vi "Glyph_MouseDown.vi"(6 "Double Click":bool, 8 "error in":errorcluster, 9 "Coords":T5, 10 "CtlRef":refnum<vi>, 11 "Data in":T1={"Class"={"Ants"=refnum, "Layer"=refnum, "Templates"=refnum, "Icon"=refnum, "Glyph"=refnum, "Settings"=refnum, "Tools"=refnum}, "Ref"={"Add Layer"=refnum, "Remove Layer"=refnum, "Line Text"=[], "Body Text Spec"=refnum, "DNL_Font"=refnum, "glyph path str"=refnum, "templates path str"=refnum, "Arrow Up"=refnum, "Arrow Down"=refnum, "IE VI Ref"=refnum, "Glyphs tree"=refnum, "Templates tree"=refnum, "Layer Icon Text"=refnum, "Layer Template"=refnum, "Body Text"=refnum, "Search Templates"=refnum, "TextMarker"=refnum, "Tab Control"=refnum, "Search Glyphs"=refnum, "Line Color"=refnum, "DNL_Glyphs []"=refnum, "Fill Color"=refnum, "Tools"=refnum, "Icon"=refnum, "Preview"=refnum, "Ants"=refnum, "Terminals"=refnum, "menu reference"=refnum, "LayerNames"=[], "GlyphLoadAnimation"=refnum, "TemplateLoadAnimation"=refnum, "refreshGlyphs"=refnum, "refreshTemplates"=refnum}, "Support"={"AntsRect"={"left"=0, "top"=0, "right"=0, "bottom"=0}, "Mouse Move Coords"={"Horizontal"=0, "Vertical"=0}, "Mouse Down Coords"={"Horizontal"=0, "Vertical"=0}, "Temp Coord"={"Horizontal"=0, "Vertical"=0}, "Action"=enum."Default", "Edge Color"=4914962, "Fill Color"=16860, "Mouse Down?"=FALSE, "Draft Mode?"=FALSE, "Temp Icon"=bytes[3102], "CTRL Pressed"=FALSE, "Move Selection?"=FALSE, "AntsRect Orig"={"left"=0, "top"=0, "right"=0, "bottom"=0}, "Text"="", "TM Set?"=FALSE, "Mouse inside icon?"=FALSE, "Tool (old value)"=0, "Pencil Move Color"=0, "Swap Colors?"=FALSE, "Shift pressed?"=FALSE}}) -> (0 "error out":errorcluster, 3 "Data out":T1={"Class"={"Ants"=refnum, "Layer"=refnum, "Templates"=refnum, "Icon"=refnum, "Glyph"=refnum, "Settings"=refnum, "Tools"=refnum}, "Ref"={"Add Layer"=refnum, "Remove Layer"=refnum, "Line Text"=[], "Body Text Spec"=refnum, "DNL_Font"=refnum, "glyph path str"=refnum, "templates path str"=refnum, "Arrow Up"=refnum, "Arrow Down"=refnum, "IE VI Ref"=refnum, "Glyphs tree"=refnum, "Templates tree"=refnum, "Layer Icon Text"=refnum, "Layer Template"=refnum, "Body Text"=refnum, "Search Templates"=refnum, "TextMarker"=refnum, "Tab Control"=refnum, "Search Glyphs"=refnum, "Line Color"=refnum, "DNL_Glyphs []"=refnum, "Fill Color"=refnum, "Tools"=refnum, "Icon"=refnum, "Preview"=refnum, "Ants"=refnum, "Terminals"=refnum, "menu reference"=refnum, "LayerNames"=[], "GlyphLoadAnimation"=refnum, "TemplateLoadAnimation"=refnum, "refreshGlyphs"=refnum, "refreshTemplates"=refnum}, "Support"={"AntsRect"={"left"=0, "top"=0, "right"=0, "bottom"=0}, "Mouse Move Coords"={"Horizontal"=0, "Vertical"=0}, "Mouse Down Coords"={"Horizontal"=0, "Vertical"=0}, "Temp Coord"={"Horizontal"=0, "Vertical"=0}, "Action"=enum."Default", "Edge Color"=4914962, "Fill Color"=16860, "Mouse Down?"=FALSE, "Draft Mode?"=FALSE, "Temp Icon"=bytes[3102], "CTRL Pressed"=FALSE, "Move Selection?"=FALSE, "AntsRect Orig"={"left"=0, "top"=0, "right"=0, "bottom"=0}, "Text"="", "TM Set?"=FALSE, "Mouse inside icon?"=FALSE, "Tool (old value)"=0, "Pencil Move Color"=0, "Swap Colors?"=FALSE, "Shift pressed?"=FALSE}})   [LabVIEW 2021]
uses:
  <vilib>/LabVIEW Icon API/lv_icon/Controls/Graphic.ctl
  <vilib>/Utility/miscctls.llb/LVPoint32TypeDef.ctl
  <resource>/plugins/NIIconEditor/Controls/Global Data.ctl
  <resource>/plugins/NIIconEditor/Class/Ants/Ants.lvclass
  <resource>/plugins/NIIconEditor/Class/FakedArray/FakedArray.lvclass
  <vilib>/LabVIEW Icon API/lv_icon/Classes/Icon/Icon.lvclass
  <resource>/plugins/NIIconEditor/Class/Icon Library/Glyph.lvclass
  <resource>/plugins/NIIconEditor/Class/Settings/Settings.lvclass
  <resource>/plugins/NIIconEditor/Class/Tools/Tools Paint.lvclass
  <resource>/plugins/NIIconEditor/Controls/IE Classes.ctl
  <resource>/plugins/NIIconEditor/Controls/References Cluster.ctl
  <resource>/plugins/NIIconEditor/Controls/SupportClass.ctl
  <resource>/plugins/NIIconEditor/Controls/SupportClass_Action.ctl
  <vilib>/LabVIEW Icon API/lv_icon/Controls/IEColor.ctl
  <resource>/plugins/NIIconEditor/Controls/Tools.ctl
  <vilib>/LabVIEW Icon API/lv_icon/lv_icon.lvlib
panel:
  in  "Path & Icon 2":T8
  in  "Path & Icon":T8
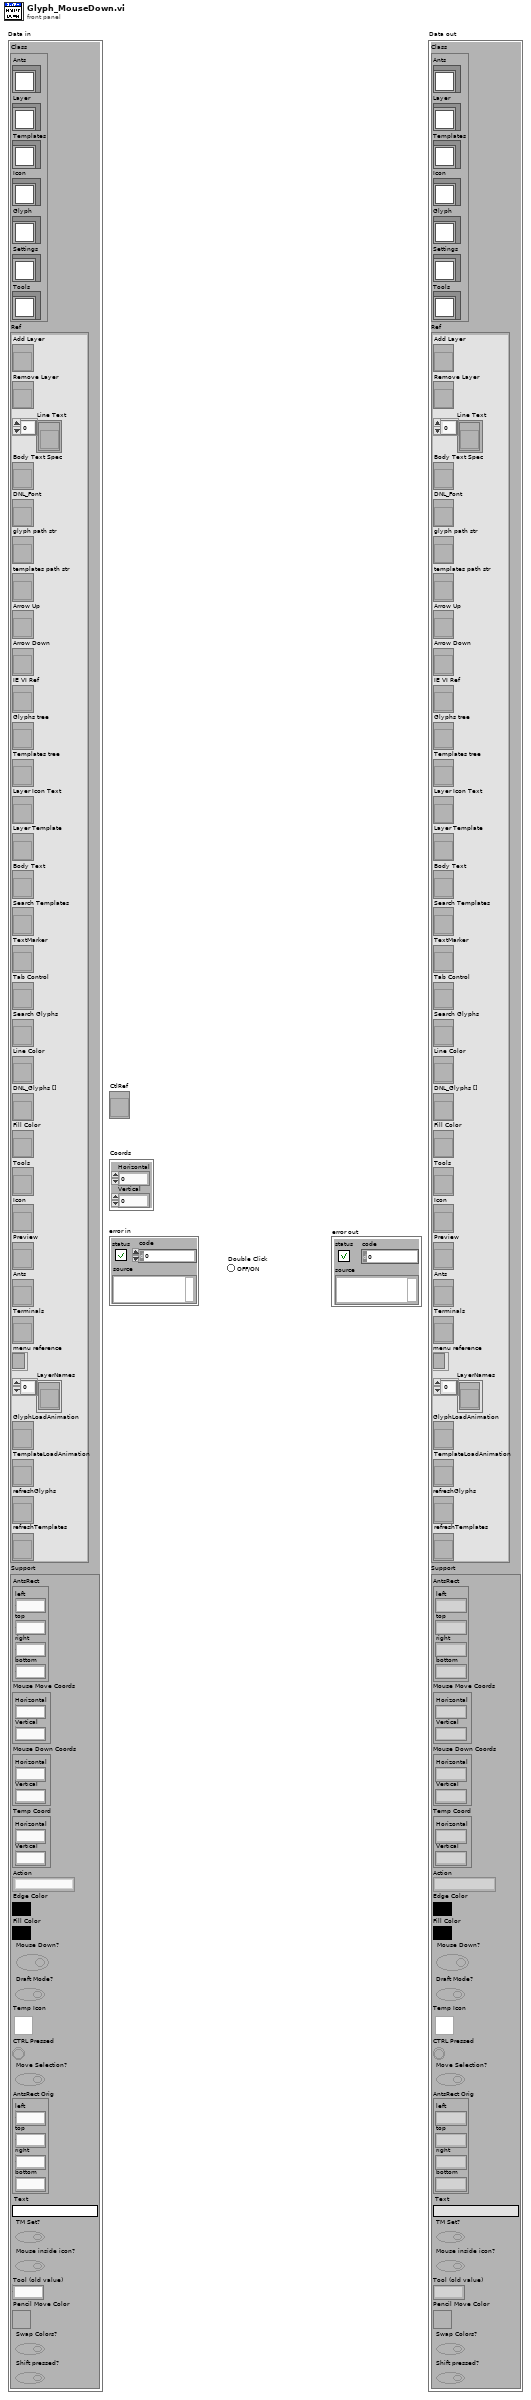
[diagram p1: front panel]
types:
  T1 = typedef "lv_icon.lvlib/Global Data.ctl" = cluster{"Class":T2, "Ref":T3, "Support":T4}
  T2 = typedef "IE Classes.ctl" = cluster{"Ants":refnum<class "Ants.lvclass">, "Layer":refnum<class "FakedArray.lvclass">, "Templates":refnum<class "FakedArray.lvclass">, "Icon":refnum<class "Icon.lvclass">, "Glyph":refnum<class "Glyph.lvclass">, "Settings":refnum<class "Settings.lvclass">, "Tools":refnum<class "Tools Paint.lvclass">}
  T3 = typedef "lv_icon.lvlib/References Cluster.ctl" = cluster{"Add Layer":refnum<vi>, "Remove Layer":refnum<vi>, "Line Text":refnum<vi>[], "Body Text Spec":refnum<vi>, "DNL_Font":refnum<vi>, "glyph path str":refnum<vi>, "templates path str":refnum<vi>, "Arrow Up":refnum<vi>, "Arrow Down":refnum<vi>, "IE VI Ref":refnum<vi>, "Glyphs tree":refnum<vi>, "Templates tree":refnum<vi>, "Layer Icon Text":refnum<vi>, "Layer Template":refnum<vi>, "Body Text":refnum<vi>, "Search Templates":refnum<vi>, "TextMarker":refnum<vi>, "Tab Control":refnum<vi>, "Search Glyphs":refnum<vi>, "Line Color":refnum<vi>, "DNL_Glyphs []":refnum<vi>, "Fill Color":refnum<vi>, "Tools":refnum<vi>, "Icon":refnum<vi>, "Preview":refnum<vi>, "Ants":refnum<vi>, "Terminals":refnum<vi>, "menu reference":refnum<k9>, "LayerNames":refnum<vi>[], "GlyphLoadAnimation":refnum<vi>, "TemplateLoadAnimation":refnum<vi>, "refreshGlyphs":refnum<vi>, "refreshTemplates":refnum<vi>}
  T4 = typedef "SupportClass.ctl" = cluster{"AntsRect":cluster{"left":i16, "top":i16, "right":i16, "bottom":i16}, "Mouse Move Coords":T5, "Mouse Down Coords":T5, "Temp Coord":T5, "Action":T6, "Edge Color":T7, "Fill Color":T7, "Mouse Down?":bool, "Draft Mode?":bool, "Temp Icon":picture, "CTRL Pressed":bool, "Move Selection?":bool, "AntsRect Orig":cluster{"left":i16, "top":i16, "right":i16, "bottom":i16}, "Text":string, "TM Set?":bool, "Mouse inside icon?":bool, "Tool (old value)":u32, "Pencil Move Color":u32, "Swap Colors?":bool, "Shift pressed?":bool}
  T5 = typedef "LVPoint32TypeDef.ctl" = cluster{"Horizontal":i32, "Vertical":i32}
  T6 = typedef "SupportClass_Action.ctl" = enum16{"Default", "Move Selection", "Glyph Library", "Tool"}
  T7 = typedef "IEColor.ctl" = u32
  T8 = typedef "Graphic.ctl" = cluster{"Rectangle":cluster{"left":i16, "top":i16, "right":i16, "bottom":i16}, "Path":path, "Image":picture, "Filter":string, "FileName":string}
  T9 = typedef "Tools.ctl" = enum32{"Pencil", "Line", "Dropper", "Fill", "Rectangle", "Filled Rectangle", "Ellipse", "Filled Ellipse", "Eraser", "Text", "Select", "Move"}
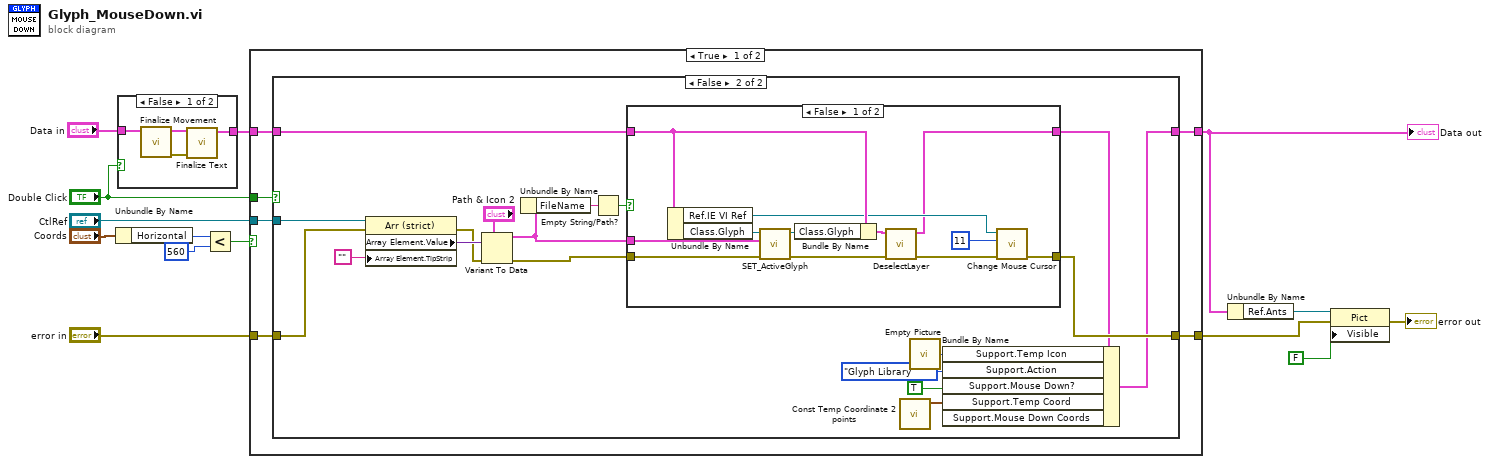
[diagram p0: block diagram]
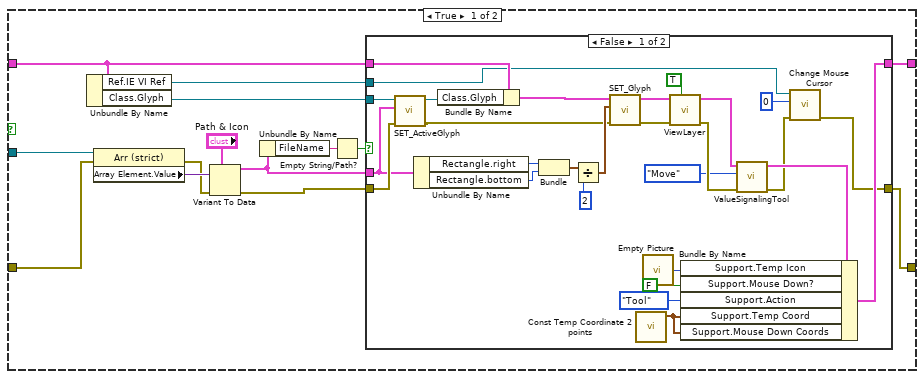
[diagram p3: hidden frame]
diagram:
  n1 = Unbundle By Name("Coords") -> ("Horizontal"=w6:i32)
  n2 = case shown="False" "Double Click" {
    tunnel: "Data in" -> [w17 w19]
    tunnel: [w15 w19] -> w4
    frame False {
      n3 = call <resource>:"Finalize Movement.vi"("Data in"=w17) -> ("error out"=w18:errorcluster, "Data out"=w16:T1)  [unwired: 2 in, 7 out]
      n4 = call <resource>:"Finalize Text.vi"("error in (no error)"=w18, "Data in"=w16) -> ("Data out"=w15:T1)  [unwired: 9 out]
    }
    frame True {
    }
  }
  n5 = Less?(x=w6, y=560 ("x")) -> (x < y?=w8:bool)
  n6 = case shown="True" w8 {
    tunnel: "CtlRef" -> [w25 _]
    tunnel: "error in" -> [w24 w103]
    tunnel: [w23 w103] -> w1
    tunnel: "Double Click" -> [w22 _]
    tunnel: w4 -> [w21 w102]
    tunnel: [w20 w102] -> w2
    frame True {
      n7 = case shown="False" w22 {
        tunnel: w25 -> [w39 w87]
        tunnel: w24 -> [w34 w83]
        tunnel: [w29 w77] -> w23
        tunnel: w21 -> [w32 w75]
        tunnel: [w31 w73] -> w20
        frame True {
          n8 = Unbundle By Name(w32) -> ("Ref.IE VI Ref"=w30:refnum<vi>, "Class.Glyph"=w33:refnum<class "Glyph.lvclass">)
          n9 = property class="Arr (strict)"(reference=w39, error in=w34) -> (error out=w37:errorcluster, "Array Element.Value"=w38:variant)  [unwired: 1 out]
          n10 = Variant To Data(error in=w37, type="Path & Icon", Variant=w38) -> (data=w27:T8, error out=w35:errorcluster)
          n11 = Unbundle By Name(w27) -> ("FileName"=w28:string)
          n12 = Empty String/Path?(string/path=w28) -> (empty?=w26:bool)
          n13 = case shown="False" w26 {
            tunnel: w35 -> [w67 w68]
            tunnel: w33 -> [w54 _]
            tunnel: w32 -> [w51 w69]
            tunnel: [w50 w69] -> w31
            tunnel: w30 -> [w43 _]
            tunnel: [w41 w68] -> w29
            tunnel: w27 -> [w40 _]
            frame False {
              n14 = call-dynamic "SET_ActiveGlyph.vi"("error in (no error)"=w67, "Active Glyph"=w40, "Glyph in"=w54) -> ("error out"=w52:errorcluster, "Glyph out"=w53:refnum<class "Glyph.lvclass">)  [unwired: 7 out]
              n15 = Unbundle By Name(w40) -> ("Rectangle.right"=w66:i16, "Rectangle.bottom"=w65:i16)
              n16 = Bundle By Name(cluster=w51, "Class.Glyph"=w53) -> (w49:T1)
              n17 = Bundle("right"=w66, "bottom"=w65) -> (w64:cluster{"right":i16, "bottom":i16})  [unwired: 1 out]
              n18 = Divide(x=w64, y=2) -> (x/y=w62:cluster{"right":dbl, "bottom":dbl})
              n19 = call <resource>:"SET_Glyph.vi"("error in"=w52, "Coordinates"=w62, "Data in"=w49) -> ("error out"=w56:errorcluster, "Data out"=w48:T1)  [unwired: 7 out]
              n20 = call <resource>:"Const Temp Coordinate 2 points.vi"() -> ("Const Temp Coordinate"=w58:T5)  [unwired: 11 out]
              n21 = call "Empty Picture"() -> ("empty picture"=w59:picture)
              n22 = call <resource>:"ViewLayer.vi"("Add to Undo?"=TRUE, "error in (no error)"=w56, "Data in"=w48) -> ("error out"=w55:errorcluster, "Data out"=w46:T1)  [unwired: 2 in, 5 out]
              n23 = call <resource>:"ValueSignalingTool.vi"("error in (no error)"=w55, "Tools"=Tools."Move", "Data in"=w46) -> ("error out"=w42:errorcluster, "Data out"=w45:T1)  [unwired: 7 out]
              n24 = Bundle By Name(cluster=w45, "Support.Temp Icon"=w59, "Support.Mouse Down?"=FALSE ("Mouse Down?"), "Support.Action"=SupportClass_Action."Tool" ("Action"), "Support.Temp Coord"=w58, "Support.Mouse Down Coords"=w58) -> (w50:T1)
              n25 = call <resource>:"Change Mouse Cursor.vi"("error in (no error)"=w42, "icon"=u16 0, "VI reference (current VI)"=w43) -> ("error out"=w41:errorcluster)  [unwired: 8 out]
            }
            frame True {
            }
          }
        }
        frame False {
          n26 = property class="Arr (strict)"(reference=w87, error in=w83, "Array Element.TipStrip"="") -> (error out=w85:errorcluster, "Array Element.Value"=w86:variant)  [unwired: 1 out]
          n27 = Variant To Data(error in=w85, type="Path & Icon 2", Variant=w86) -> (data=w72:T8, error out=w76:errorcluster)
          n28 = Unbundle By Name(w72) -> ("FileName"=w70:string)
          n29 = Empty String/Path?(string/path=w70) -> (empty?=w71:bool)
          n30 = case shown="False" w71 {
            tunnel: [w98 w101] -> w77
            tunnel: w76 -> [w97 w101]
            tunnel: w75 -> [w95 w100]
            tunnel: [w89 w100] -> w74
            tunnel: w72 -> [w88 _]
            frame False {
              n31 = Unbundle By Name(w95) -> ("Ref.IE VI Ref"=w94:refnum<vi>, "Class.Glyph"=w92:refnum<class "Glyph.lvclass">)
              n32 = call-dynamic "SET_ActiveGlyph.vi"("error in (no error)"=w97, "Active Glyph"=w88, "Glyph in"=w92) -> ("error out"=w91:errorcluster, "Glyph out"=w93:refnum<class "Glyph.lvclass">)  [unwired: 7 out]
              n33 = Bundle By Name(cluster=w95, "Class.Glyph"=w93) -> (w90:T1)
              n34 = call <resource>:"DeselectLayer.vi"("error in (no error)"=w91, "Data in"=w90) -> ("error out"=w99:errorcluster, "Data out"=w89:T1)  [unwired: 8 out]
              n35 = call <resource>:"Change Mouse Cursor.vi"("error in (no error)"=w99, "icon"=u16 11, "VI reference (current VI)"=w94) -> ("error out"=w98:errorcluster)  [unwired: 8 out]
            }
            frame True {
            }
          }
          n36 = call <resource>:"Const Temp Coordinate 2 points.vi"() -> ("Const Temp Coordinate"=w79:T5)  [unwired: 11 out]
          n37 = call "Empty Picture"() -> ("empty picture"=w80:picture)
          n38 = Bundle By Name(cluster=w74, "Support.Temp Icon"=w80, "Support.Action"=SupportClass_Action."Glyph Library" ("Action"), "Support.Mouse Down?"=TRUE ("Mouse Down?"), "Support.Temp Coord"=w79, "Support.Mouse Down Coords"=w79) -> (w73:T1)
        }
      }
    }
    frame False {
    }
  }
  "Data out" <- w2
  n39 = Unbundle By Name(w2) -> ("Ref.Ants"=w9:refnum<vi>)
  n40 = property class="Pict"(reference=w9, error in=w1, "Visible"=FALSE) -> (error out=→"error out":errorcluster)  [unwired: 1 out]
